vi "Sets_Intersect(VI-REF).vi"(8 "error in (no error)":errorcluster caption="错误输入（无错误）", 10 "输入数组B":refnum<vi>[](array[refnum]), 11 "输入数组A":refnum<vi>[](array[refnum])) -> (0 "error out":errorcluster caption="错误输出", 3 "输出数组C":refnum<vi>[](array[refnum]))   [LabVIEW 2011]
uses:
  Sets_Unique(VI-REF).vi
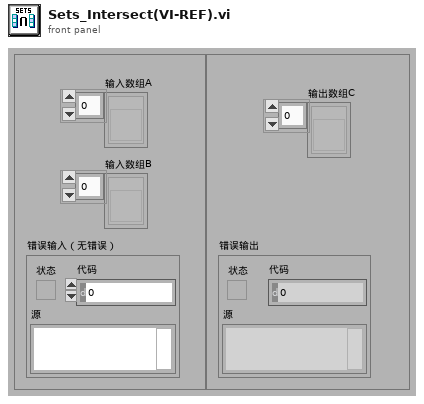
[diagram p1: front panel]
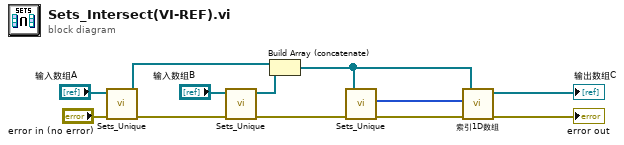
[diagram p0: block diagram]
diagram:
  n1 = call-poly "Sets_Unique.vi"("error in (no error)"="error in (no error)", "输入数组"="输入数组A") -> ("error out"=w10:errorcluster, "输出数组"=w4:refnum<vi>[])  [unwired: 7 in, 1 out]
  n2 = call-poly "Sets_Unique.vi"("error in (no error)"=w10, "输入数组"="输入数组B") -> ("error out"=w11:errorcluster, "输出数组"=w3:refnum<vi>[])  [unwired: 7 in, 1 out]
  n3 = Build Array (concatenate)(w4, w3) -> (w5:refnum<vi>[])
  n4 = call-poly "Sets_Unique.vi"("error in (no error)"=w11, "输入数组"=w5) -> ("error out"=w7:errorcluster, "已删除元素索引"=w6:i32[])  [unwired: 7 in, 1 out]
  n5 = call-poly "索引1D数组.vi"("error in (no error)"=w7, "索引"=w6, "输入数组"=w5) -> ("error out"=→"error out":errorcluster, "元素"=→"输出数组C":refnum<vi>[])  [unwired: 7 in]
